vi "_10_Sample_qsns_03[13].vi"() -> ()   [LabVIEW 2020]
panel:
  out "appended array":i32[][](array[numeric])
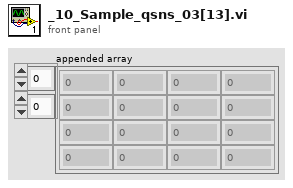
[diagram p1: front panel]
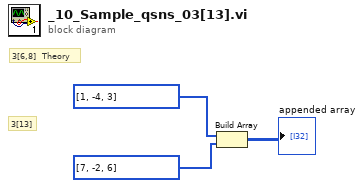
[diagram p0: block diagram]
diagram:
  # "3[6,8]  Theory"
  # "3[13]"
  n1 = Build Array "Build Array"(i32[] [1, -4, 3], i32[] [7, -2, 6]) -> (→"appended array":i32[][])
